vi "FormatAlarmString.vi"(0 "Timestamp_sec":dbl, 5 "ChannelIndex":i32, 7 "ChannelName":string, 9 "AlarmTableIn":string[][](array[string])) -> (10 "AlarmTableOut":string[][](array[string]))   [LabVIEW 2018]
doc: "Format this alarm into a row of strings and append it to the AlarmTableIn as a new row."
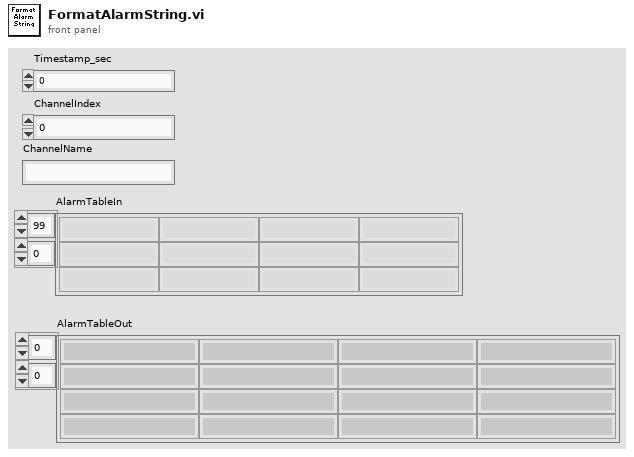
[diagram p1: front panel]
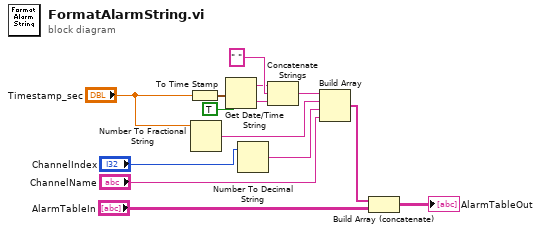
[diagram p0: block diagram]
diagram:
  n1 = To Time Stamp(1:"Timestamp_sec") -> (0:w4:timestamp)
  n2 = Number To Fractional String(number="Timestamp_sec") -> (F-format string=w3:string)  [unwired: 3 in]
  n3 = Get Date/Time String(seconds (now)=w4, want seconds? (F)=TRUE) -> (date string=w6:string, time string=w7:string)  [unwired: 1 in]
  n4 = Number To Decimal String(number="ChannelIndex") -> (decimal integer string=w9:string)  [unwired: 1 in]
  n5 = Concatenate Strings(w6, " " ("string"), w7) -> (w2:string)
  n6 = Build Array(w2, w3, w9, "ChannelName") -> (w10:string[])
  n7 = Build Array (concatenate)(w10, "AlarmTableIn") -> (→"AlarmTableOut":string[][])
